vi "Experiment-2-4-1.vi"() -> ()   [LabVIEW 2014]
panel:
  out "y":dbl
  in  "x":dbl
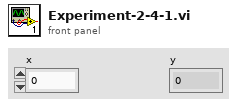
[diagram p1: front panel]
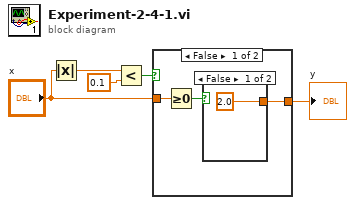
[diagram p0: block diagram]
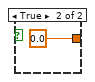
[diagram p2: hidden frame]
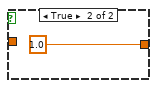
[diagram p3: hidden frame]
diagram:
  n1 = Absolute Value(x="x") -> (abs(x)=w5:dbl)
  n2 = Less?(x=w5, y=0.1) -> (x < y?=w4:bool)
  n3 = case shown="False" w4 {
    tunnel: [w6 1.0] -> w2
    tunnel: "x" -> [w8 _]
    frame False {
      n4 = Greater Or Equal To 0?(x=w8) -> (x >= 0?=w7:bool)
      n5 = case shown="False" w7 {
        tunnel: [2.0 0.0] -> w6
        frame False {
        }
        frame True {
        }
      }
    }
    frame True {
    }
  }
  "y" <- w2
